vi "Setup4 Config.vi"(7 "Ring":u16(ring) items=["Read from ini files (to cluster Params)", "Write to ini file (from cluster Params)", "Copy ini file to new Path", "Create new lookup table by default value"], 8 "error in (no error)":errorcluster, 9 "Copy path":path, 10 "Config file to read/write":path, 11 "Params in":T2={"TaskIDs"={"DAQ tasks"={"Px taskID"=0, "Py taskID"=0, "Pz taskID"=0, "AOM taskID"=0, "Clock taskID"=0, "AI taskID"=0}, "DVEHandle"=refnum}, "Manual Control"={"Rotation Control"={"Phase"=0.0, "A amp (0-120)"=75.0, "B amp (0-120)"=53.3, "mean freq  [MHz]\ndefault 39.99"=40.0, "freq difference [Hz]"=2.0, "Enable A"=TRUE, "Enable B"=TRUE}, "X piezo\n [nm]"=0.0, "Y peizo\n [nm]"=0.0, "trap height\n [nm]"=5.012658227848101, "AOM0 \nPower"=0.2}, "Piezo Calibr"={"Px2Vx(AO)"=nan, "Py2Vy(AO)"=nan, "Pz2Vz(AO)"=nan, "Min Px"=nan, "Min Py"=nan, "Min Pz"=nan, "Max Px"=nan, "Max Py"=nan, "Max Pz"=nan, "Vx0 (V)"=nan, "Vy0 (V)"=nan, "Vz0 (V)"=nan}, "Instrument Calibr"={"Angular compensation coeffs"=[], "TetherCenter"={"TrapX_AO 0 [nm]"=nan, "TrapY_AO 0 [nm]"=nan, "TrapZ_AO 0 [nm]"=nan}, "XYZsignal baseline"={"Xsignal0"=nan, "Ysignal0"=nan, "Zsignal0"=nan, "Zsig slope"=nan, "Z bead0"=nan}, "S and P to Vs0"={"Vs0/P"=1.0, "Vs0/S"=1.0}, "Psi"=0.0, "ePS:eRL drift correlation"={"Interc P"=nan, "Slope P"=nan, "Interc S"=nan, "Slope S"=nan}, "Current piezo volt AO"={"Vpx_AO [V]"=nan, "Vpy_AO [V]"=nan, "Vpz_AO [V]"=nan}}, "Cylinder Calibr"={"ZStiff"=nan, "Zsens"=nan, "AngStiff"=nan, "XStiff"=nan, "Xsens"=nan, "MaxEllip"=nan, "YStiff"=nan, "Ysens"=nan, "FocalShift"=nan, "Sfz"=nan, "1/Sz"=nan, "Stau"=nan, "Sfx"=nan, "1/Sx"=nan, "1/Sang"=nan, "Sfy"=nan, "1/Sy"=nan, "1/focal"=nan, "ZsignalHeightDependence (1/nm)"=0.0}, "DAQParams"={"Buffer size"=nan, "Scanning rate"=nan, "Average"=nan, "Sampling rate"=nan, "set dt"=nan}, "DAQ channel offsets"={"A0 [V]"=0.0, "D0 [V]"=0.0, "P0  [V]"=0.0, "S0 [V]"=0.0, "L0 [V]"=0.0, "R0 [V]"=0.0, "Vpx0 [V]"=0.0, "Vpy0 [V]"=0.0, "Vpz0 [V]"=0.0, "Vsum0 [V]"=0.0, "Vpx_AO0 [V]"=0.0, "Vpy_AO0 [V]"=0.0, "Vpz_AO0 [V]"=0.0}, "Z bead polynomial coeffs"=[nan, nan, nan, nan], "Skip button ref"=refnum, "z bead lookup table"={"z signal"=[], "z bead"=[]}, "SP->power Matrix"=[], "Ms2p"=[], "Mp2s"=[], "Polynomial coeff V_px,y,z 2 position (nm)"=[]} {"Cylinder Calibr"."ZsignalHeightDependence (1/nm)" format="%.4e"; "Instrument Calibr"."Psi" format="%#_2f"; "Manual Control"."Y peizo\n [nm]" step=100.0 scale=0.0..30000.0; "Manual Control"."AOM0 \nPower" scale=0.0..1.0; "Manual Control"."X piezo\n [nm]" step=100.0 scale=0.0..30000.0; "Manual Control"."Rotation Control"."mean freq  [MHz]\ndefault 39.99" min=0.0 step=0.01; "Manual Control"."Rotation Control"."B amp (0-120)" min=0.0 max=120.0 step=0.1 format="%.1f"; "Manual Control"."Rotation Control"."A amp (0-120)" min=0.0 max=120.0 step=0.1 format="%.1f"; "Manual Control"."Rotation Control"."Phase" scale=0.0..360.0; "Manual Control"."trap height\n [nm]" scale=1000.0..7500.0; "TaskIDs"."DAQ tasks"."Px taskID" format="%x"; "TaskIDs"."DAQ tasks"."Py taskID" format="%x"; "TaskIDs"."DAQ tasks"."Pz taskID" format="%x"; "TaskIDs"."DAQ tasks"."AOM taskID" format="%x"; "TaskIDs"."DAQ tasks"."Clock taskID" format="%x"; "TaskIDs"."DAQ tasks"."AI taskID" format="%x"}) -> (0 "error out":errorcluster, 2 "file path out":path, 3 "Params out":T2={"TaskIDs"={"DAQ tasks"={"Px taskID"=0, "Py taskID"=0, "Pz taskID"=0, "AOM taskID"=0, "Clock taskID"=0, "AI taskID"=0}, "DVEHandle"=refnum}, "Manual Control"={"Rotation Control"={"Phase"=0.0, "A amp (0-120)"=75.0, "B amp (0-120)"=53.3, "mean freq  [MHz]\ndefault 39.99"=40.0, "freq difference [Hz]"=2.0, "Enable A"=TRUE, "Enable B"=TRUE}, "X piezo\n [nm]"=0.0, "Y peizo\n [nm]"=0.0, "trap height\n [nm]"=5.012658227848101, "AOM0 \nPower"=0.2}, "Piezo Calibr"={"Px2Vx(AO)"=nan, "Py2Vy(AO)"=nan, "Pz2Vz(AO)"=nan, "Min Px"=nan, "Min Py"=nan, "Min Pz"=nan, "Max Px"=nan, "Max Py"=nan, "Max Pz"=nan, "Vx0 (V)"=nan, "Vy0 (V)"=nan, "Vz0 (V)"=nan}, "Instrument Calibr"={"Angular compensation coeffs"=[], "TetherCenter"={"TrapX_AO 0 [nm]"=nan, "TrapY_AO 0 [nm]"=nan, "TrapZ_AO 0 [nm]"=nan}, "XYZsignal baseline"={"Xsignal0"=nan, "Ysignal0"=nan, "Zsignal0"=nan, "Zsig slope"=nan, "Z bead0"=nan}, "S and P to Vs0"={"Vs0/P"=1.0, "Vs0/S"=1.0}, "Psi"=0.0, "ePS:eRL drift correlation"={"Interc P"=nan, "Slope P"=nan, "Interc S"=nan, "Slope S"=nan}, "Current piezo volt AO"={"Vpx_AO [V]"=nan, "Vpy_AO [V]"=nan, "Vpz_AO [V]"=nan}}, "Cylinder Calibr"={"ZStiff"=nan, "Zsens"=nan, "AngStiff"=nan, "XStiff"=nan, "Xsens"=nan, "MaxEllip"=nan, "YStiff"=nan, "Ysens"=nan, "FocalShift"=nan, "Sfz"=nan, "1/Sz"=nan, "Stau"=nan, "Sfx"=nan, "1/Sx"=nan, "1/Sang"=nan, "Sfy"=nan, "1/Sy"=nan, "1/focal"=nan, "ZsignalHeightDependence (1/nm)"=0.0}, "DAQParams"={"Buffer size"=nan, "Scanning rate"=nan, "Average"=nan, "Sampling rate"=nan, "set dt"=nan}, "DAQ channel offsets"={"A0 [V]"=0.0, "D0 [V]"=0.0, "P0  [V]"=0.0, "S0 [V]"=0.0, "L0 [V]"=0.0, "R0 [V]"=0.0, "Vpx0 [V]"=0.0, "Vpy0 [V]"=0.0, "Vpz0 [V]"=0.0, "Vsum0 [V]"=0.0, "Vpx_AO0 [V]"=0.0, "Vpy_AO0 [V]"=0.0, "Vpz_AO0 [V]"=0.0}, "Z bead polynomial coeffs"=[nan, nan, nan, nan], "Skip button ref"=refnum, "z bead lookup table"={"z signal"=[], "z bead"=[]}, "SP->power Matrix"=[], "Ms2p"=[], "Mp2s"=[], "Polynomial coeff V_px,y,z 2 position (nm)"=[]} {"Cylinder Calibr"."ZsignalHeightDependence (1/nm)" format="%.4e"; "Instrument Calibr"."Psi" format="%#_2f"; "Manual Control"."Y peizo\n [nm]" step=100.0 scale=0.0..30000.0; "Manual Control"."AOM0 \nPower" scale=0.0..1.0; "Manual Control"."X piezo\n [nm]" step=100.0 scale=0.0..30000.0; "Manual Control"."Rotation Control"."mean freq  [MHz]\ndefault 39.99" min=0.0 step=0.01; "Manual Control"."Rotation Control"."B amp (0-120)" min=0.0 max=120.0 step=0.1 format="%.1f"; "Manual Control"."Rotation Control"."A amp (0-120)" min=0.0 max=120.0 step=0.1 format="%.1f"; "Manual Control"."Rotation Control"."Phase" scale=0.0..360.0; "Manual Control"."trap height\n [nm]" scale=1000.0..7500.0; "TaskIDs"."DAQ tasks"."Px taskID" format="%x"; "TaskIDs"."DAQ tasks"."Py taskID" format="%x"; "TaskIDs"."DAQ tasks"."Pz taskID" format="%x"; "TaskIDs"."DAQ tasks"."AOM taskID" format="%x"; "TaskIDs"."DAQ tasks"."Clock taskID" format="%x"; "TaskIDs"."DAQ tasks"."AI taskID" format="%x"})   [LabVIEW 2020, in "Initialization.lvlib" / "FileManagement.lvlib"]
uses:
  FileManagement.lvlib
  Param.ctl
  ManualCtrl.ctl
  DVESetting.ctl
  CylinderCalibrNew.ctl
  SignalConversion/DAQChannelOffsets.ctl
  <vilib>/Analysis/Matrix/Datatypes/RealMatrix.ctl
  configuration file sections, keys and values.ctl
  <vilib>/Utility/config.llb/Read Key (Double).vi
  <vilib>/Utility/config.llb/Read Key (String).vi
  <vilib>/Utility/config.llb/Read Key (I32).vi
  <vilib>/Analysis/baseanly.llb/Real Inverse Matrix.vi
  <vilib>/Utility/config.llb/Write Key (Double).vi
  <vilib>/Utility/config.llb/Write Key (String).vi
  <vilib>/Utility/config.llb/NI_LVConfig.lvlib
  <vilib>/Analysis/NI_AALBase.lvlib
  Initialization.lvlib
  <vilib>/Analysis/Matrix/NI_Matrix.lvlib
  SignalConversion/SignalConverson.lvlib
panel:
  in  "Piezo sensor conversion coeffs key":string="AI2p"
  out "transposed array":dbl[][](array[numeric])
  out "look up table check":string
  in  "configuration file sections, keys and values":T1={"Section 1"="Trap and cylinder calibration", "Keys of Section 1"=["Kz, pN/nm/W", "Kx, pN/nm/W", "Ky, pN/nm/W", "Sz, 1/nm", "Sx, 1/nm", "Sy, 1/nm", "Kang, pNnm/rad/W", "Max ellipticity, 1", "Focal shift", "ZsignalHeightDependence, 1/nm"], "Values (read) of Section 1"=[0.468, 4.584, 4.884, 0.000564, 0.001578, 0.00166, 30700.0, 0.0204, 0.75, 6.2e-07], "Section 2"="Piezo AO calibration and settings", "Keys of Section 2"=["Vx/Px(V/nm)", "Vy/Py(V/nm)", "Vz/Pz(V/nm)", "Max Px (nm)", "Max Py (nm)", "Max Pz (nm)", "Min Px (nm)", "Min Py (nm)", "Min Pz (nm)", "Vx0 (V)", "Vy0 (V)", "Vz0 (V)"], "Values (read) of Section 2"=[0.000665, 0.000665, 0.002, 10000.0, 10000.0, 10000.0, 0.0, 0.0, 0.0, -10.0, -10.0, -10.0], "Section 3"="matrix Mp2s (3X3)", "Keys of Section 3"=["a11", "a12", "a13", "a21", "a22", "a23", "a31", "a32", "a33"], "Values (read) of Section 3"=[1.0, 0.0, 0.0, 0.0, 1.0, 0.0, 0.0, 0.198, 1.0], "Section 4"="DAQ settings", "Keys of Section 4"=["AIBufferSize", "DAQ ScanRate", "Points to average", "Samping rate"], "Values (read) of Section 4"=[100000, 10000, 20, 500], "Section 5"="PS detector signal to laser power (W) conversion matrix (2X2)", "Keys of Section 5"=["a11", "a12", "a21", "a22"], "Values (read) of Section 5"=[-0.018123, 0.000111, 4.2e-05, -0.018644], "Section 6"="Z bead vs Z signal polynomial coefficients (nm)", "Keys of Section 6"=["a0", "a1", "a2", "a3", "a4", "a5"], "Values (read) of Section 6"=[0.0, 1064.07, 1642.745, 6870.906, -346812.49, 1661133.202], "Section 7"="Z bead look up table", "Keys of Section 7"=["(Z signal, Z bead)"], "Values (read) of Section 7"=[]}
  out "succeeded in writing to ini file ?":bool
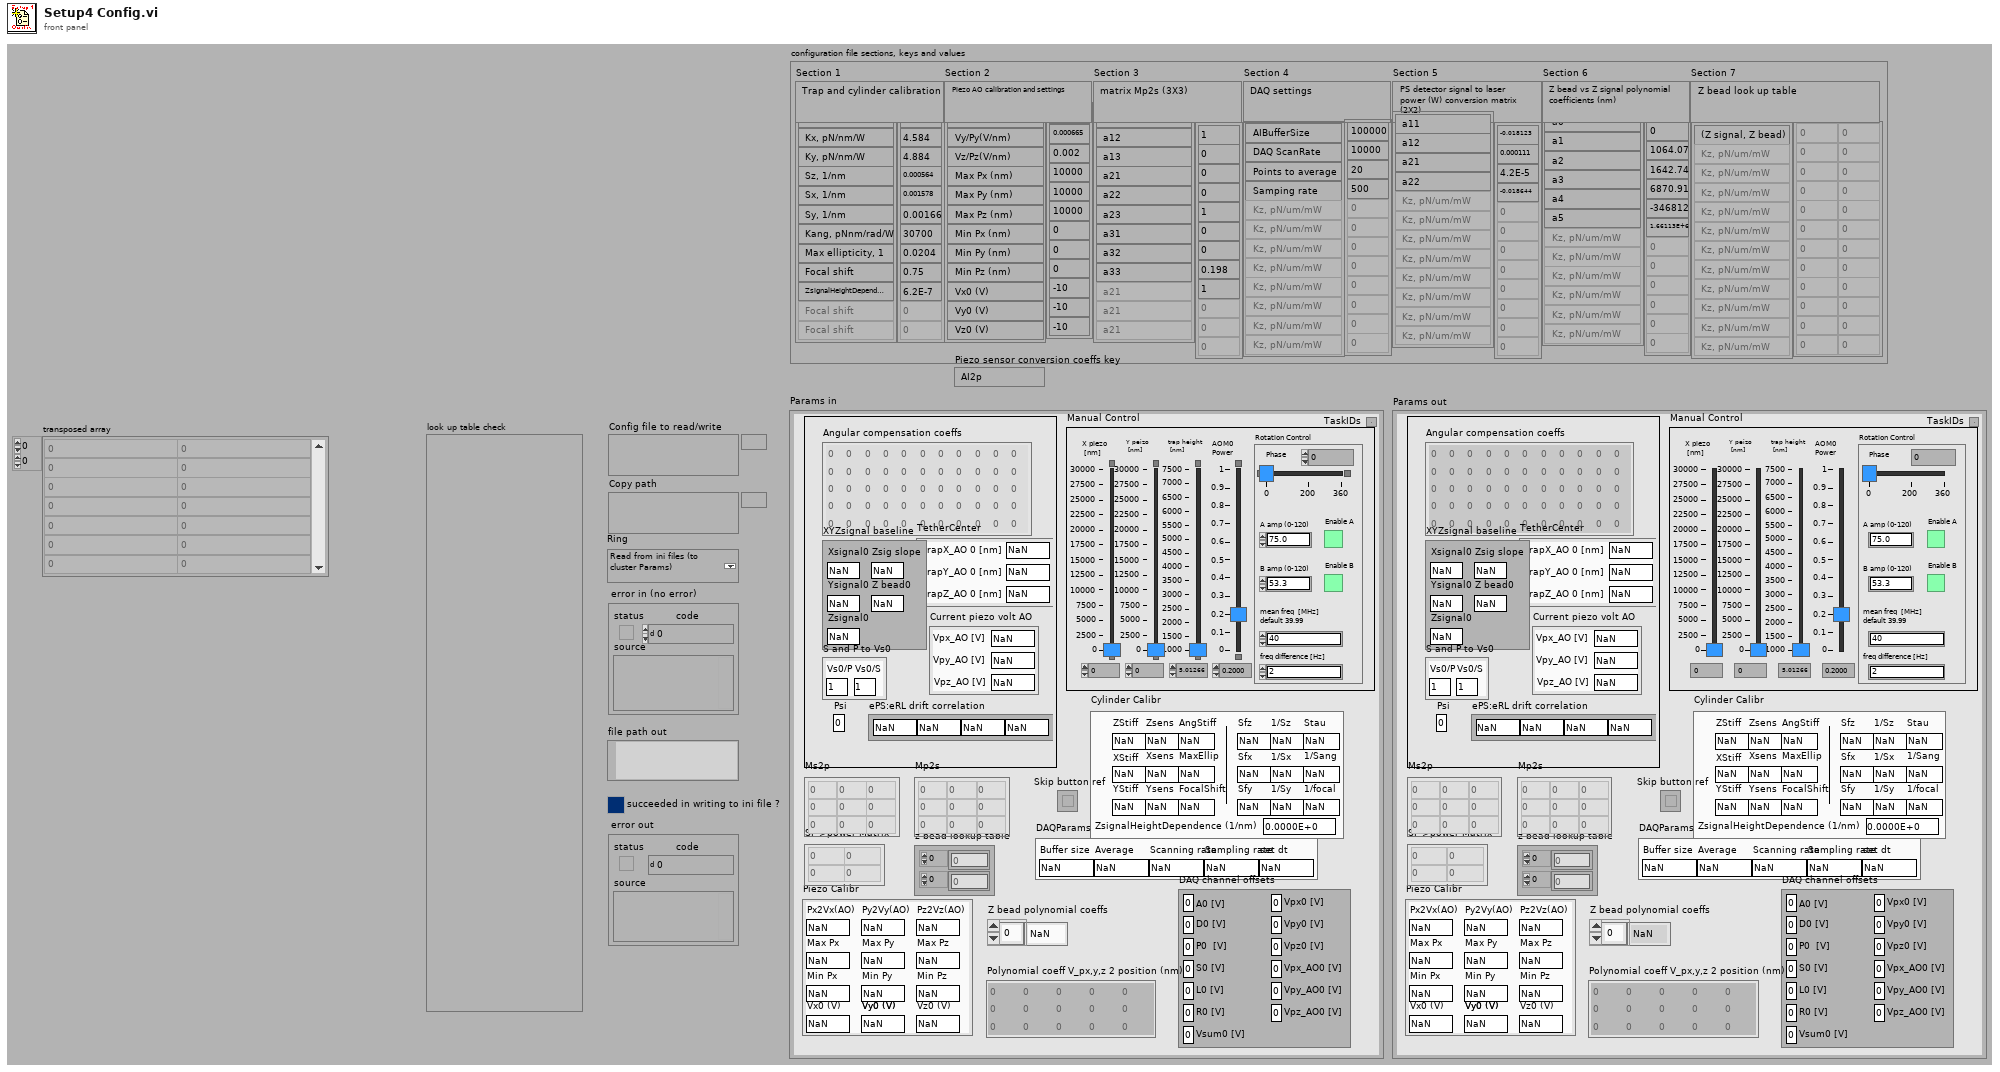
[diagram p1: front panel]
types:
  T1 = typedef "Initialization.lvlib/FileManagement.lvlib/configuration file sections, keys and values.ctl" = cluster{"Section 1":string, "Keys of Section 1":string[], "Values (read) of Section 1":dbl[], "Section 2":string, "Keys of Section 2":string[], "Values (read) of Section 2":dbl[], "Section 3":string, "Keys of Section 3":string[], "Values (read) of Section 3":dbl[], "Section 4":string, "Keys of Section 4":string[], "Values (read) of Section 4":i32[], "Section 5":string, "Keys of Section 5":string[], "Values (read) of Section 5":dbl[], "Section 6":string, "Keys of Section 6":string[], "Values (read) of Section 6":dbl[], "Section 7":string, "Keys of Section 7":string[], "Values (read) of Section 7":dbl[][]}
  T2 = typedef "Initialization.lvlib/Param.ctl" = cluster{"TaskIDs":cluster{"DAQ tasks":cluster{"Px taskID":u32, "Py taskID":u32, "Pz taskID":u32, "AOM taskID":u32, "Clock taskID":u32, "AI taskID":u32}, "DVEHandle":refnum<file>}, "Manual Control":T3, "Piezo Calibr":cluster{"Px2Vx(AO)":dbl, "Py2Vy(AO)":dbl, "Pz2Vz(AO)":dbl, "Min Px":dbl, "Min Py":dbl, "Min Pz":dbl, "Max Px":dbl, "Max Py":dbl, "Max Pz":dbl, "Vx0 (V)":dbl, "Vy0 (V)":dbl, "Vz0 (V)":dbl}, "Instrument Calibr":cluster{"Angular compensation coeffs":dbl[][], "TetherCenter":cluster{"TrapX_AO 0 [nm]":dbl, "TrapY_AO 0 [nm]":dbl, "TrapZ_AO 0 [nm]":dbl}, "XYZsignal baseline":cluster{"Xsignal0":dbl, "Ysignal0":dbl, "Zsignal0":dbl, "Zsig slope":dbl, "Z bead0":dbl}, "S and P to Vs0":cluster{"Vs0/P":dbl, "Vs0/S":dbl}, "Psi":dbl, "ePS:eRL drift correlation":cluster{"Interc P":dbl, "Slope P":dbl, "Interc S":dbl, "Slope S":dbl}, "Current piezo volt AO":cluster{"Vpx_AO [V]":dbl, "Vpy_AO [V]":dbl, "Vpz_AO [V]":dbl}}, "Cylinder Calibr":T5, "DAQParams":cluster{"Buffer size":dbl, "Scanning rate":dbl, "Average":dbl, "Sampling rate":dbl, "set dt":dbl}, "DAQ channel offsets":T6, "Z bead polynomial coeffs":dbl[], "Skip button ref":refnum<vi>, "z bead lookup table":cluster{"z signal":dbl[], "z bead":dbl[]}, "SP->power Matrix":T7, "Ms2p":T7, "Mp2s":T7, "Polynomial coeff V_px,y,z 2 position (nm)":dbl[][]}
  T3 = typedef "Initialization.lvlib/ManualCtrl.ctl" = cluster{"Rotation Control":T4, "X piezo\n [nm]":dbl, "Y peizo\n [nm]":dbl, "trap height\n [nm]":dbl, "AOM0 \nPower":dbl}
  T4 = typedef "Initialization.lvlib/DVESetting.ctl" = cluster{"Phase":dbl, "A amp (0-120)":dbl, "B amp (0-120)":dbl, "mean freq  [MHz]\ndefault 39.99":dbl, "freq difference [Hz]":dbl, "Enable A":bool, "Enable B":bool}
  T5 = typedef "Initialization.lvlib/CylinderCalibrNew.ctl" = cluster{"ZStiff":dbl, "Zsens":dbl, "AngStiff":dbl, "XStiff":dbl, "Xsens":dbl, "MaxEllip":dbl, "YStiff":dbl, "Ysens":dbl, "FocalShift":dbl, "Sfz":dbl, "1/Sz":dbl, "Stau":dbl, "Sfx":dbl, "1/Sx":dbl, "1/Sang":dbl, "Sfy":dbl, "1/Sy":dbl, "1/focal":dbl, "ZsignalHeightDependence (1/nm)":dbl}
  T6 = typedef "SignalConverson.lvlib/DAQChannelOffsets.ctl" = cluster{"A0 [V]":dbl, "D0 [V]":dbl, "P0  [V]":dbl, "S0 [V]":dbl, "L0 [V]":dbl, "R0 [V]":dbl, "Vpx0 [V]":dbl, "Vpy0 [V]":dbl, "Vpz0 [V]":dbl, "Vsum0 [V]":dbl, "Vpx_AO0 [V]":dbl, "Vpy_AO0 [V]":dbl, "Vpz_AO0 [V]":dbl}
  T7 = typedef "NI_Matrix.lvlib/RealMatrix.ctl" = dbl[][]
  T8 = typedef "NI_LVConfig.lvlib/Config Data RefNum.ctl" = refnum<k1>
  T9 = cluster{"Px2Vx(AO)":dbl, "Py2Vy(AO)":dbl, "Pz2Vz(AO)":dbl, "Min Px":dbl, "Min Py":dbl, "Min Pz":dbl, "Max Px":dbl, "Max Py":dbl, "Max Pz":dbl, "Vx0 (V)":dbl, "Vy0 (V)":dbl, "Vz0 (V)":dbl}
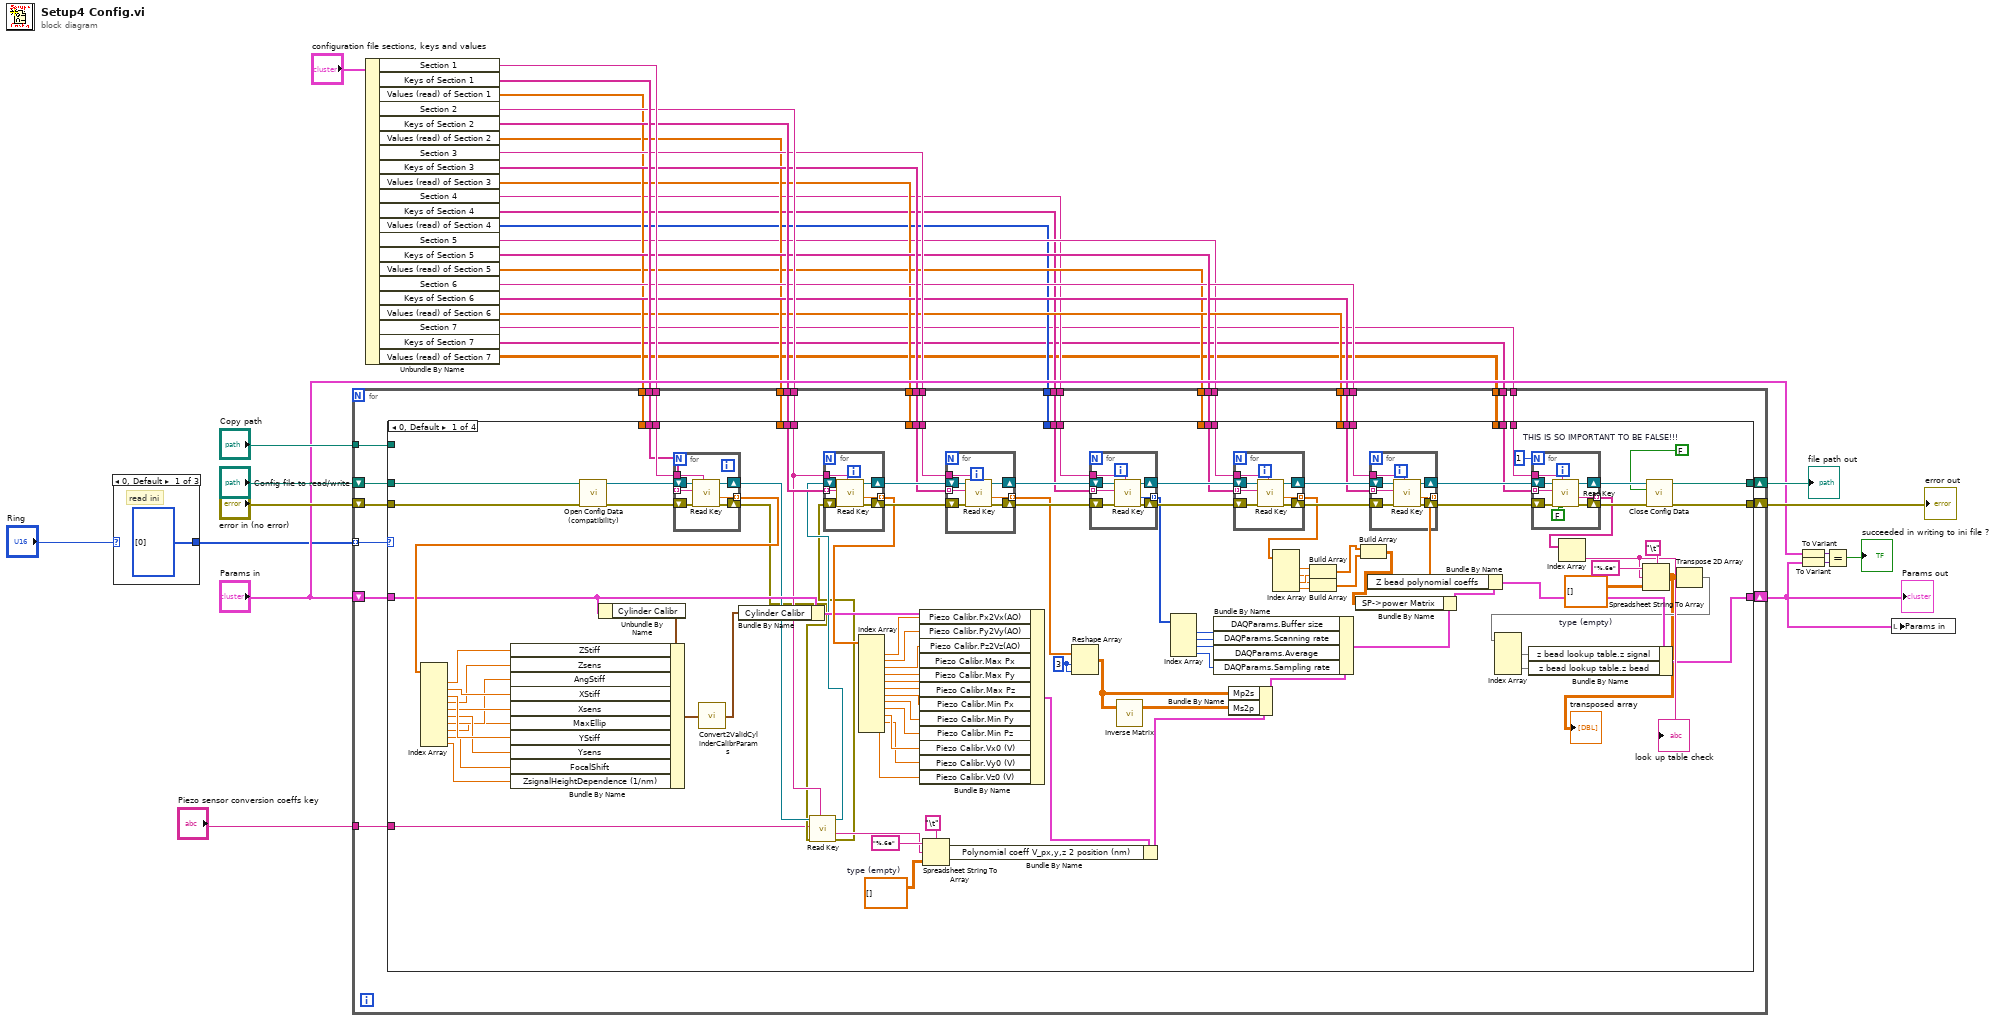
[diagram p0: block diagram]
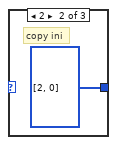
[diagram p2: hidden frame]
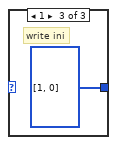
[diagram p3: hidden frame]
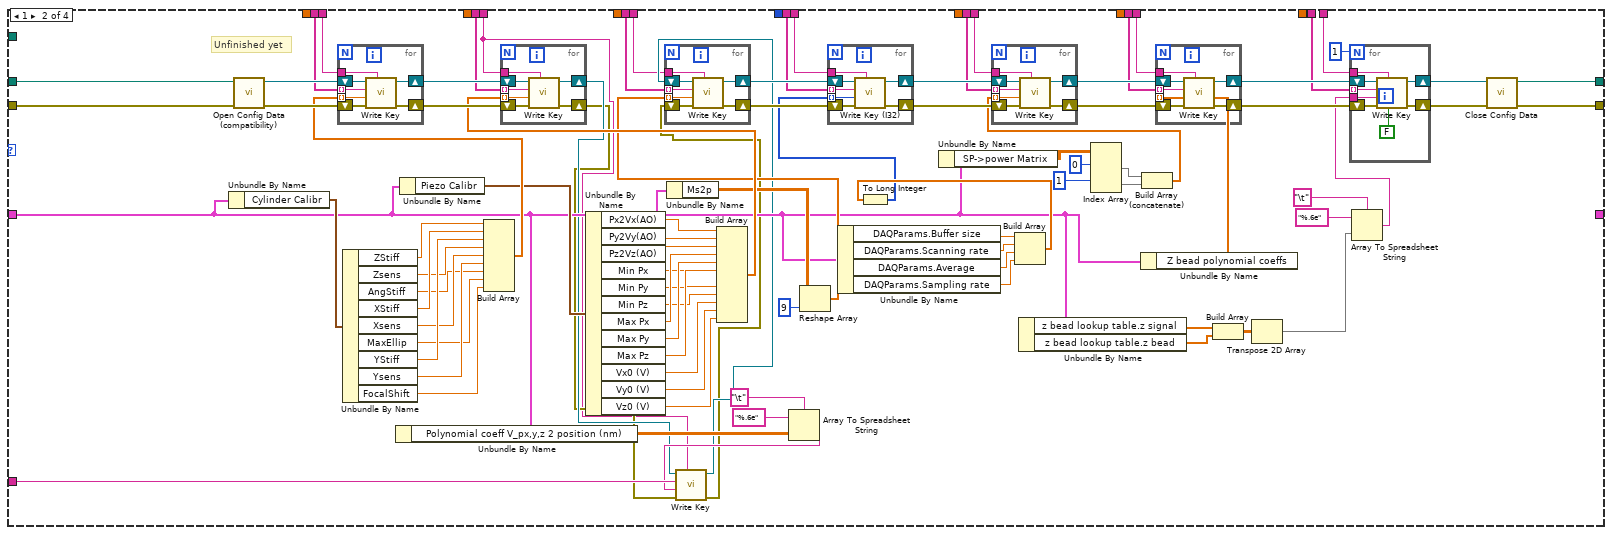
[diagram p4: hidden frame]
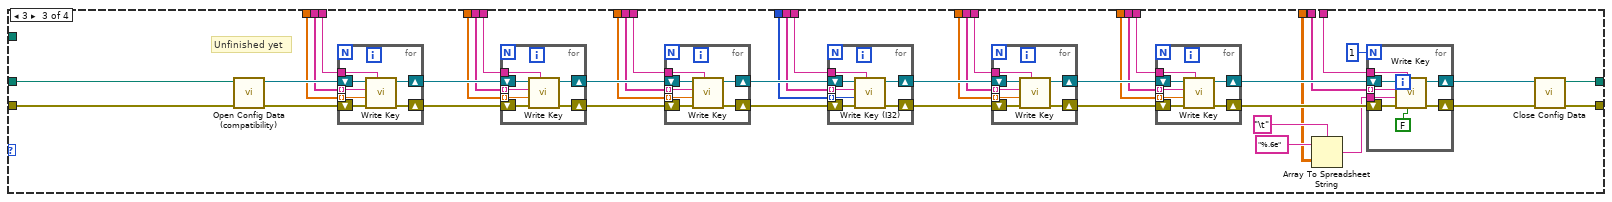
[diagram p5: hidden frame]
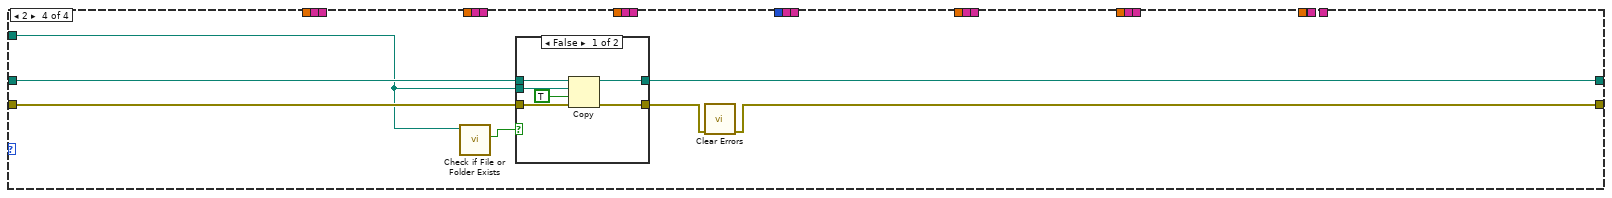
[diagram p6: hidden frame]
diagram:
  n1 = case shown="0, Default" "Ring" {
    tunnel: [i32[] [0] i32[] [2, 0] i32[] [1, 0]] -> w25
    frame 0, Default {
      # "read ini"
    }
    frame 2 {
      # "copy ini"
    }
    frame 1 {
      # "write ini"
    }
  }
  n2 = Unbundle By Name("configuration file sections, keys and values") -> ("Section 1"=w23:string, "Keys of Section 1"=w22:string[], "Values (read) of Section 1"=w14:dbl[], "Section 2"=w21:string, "Keys of Section 2"=w20:string[], "Values (read) of Section 2"=w13:dbl[], "Section 3"=w19:string, "Keys of Section 3"=w18:string[], "Values (read) of Section 3"=w12:dbl[], "Section 4"=w6:string, "Keys of Section 4"=w7:string[], "Values (read) of Section 4"=w8:i32[], "Section 5"=w9:string, "Keys of Section 5"=w17:string[], "Values (read) of Section 5"=w10:dbl[], "Section 6"=w16:string, "Keys of Section 6"=w15:string[], "Values (read) of Section 6"=w11:dbl[], "Section 7"=w5:string, "Keys of Section 7"=w4:string[], "Values (read) of Section 7"=w3:dbl[][])
  n3 = for {
    tunnel: w25 -> [w66] mode=indexing
    tunnel: w23 -> [w64]
    tunnel: w22 -> [w63]
    tunnel: w20 -> [w62]
    tunnel: w21 -> [w61]
    tunnel: w18 -> [w60]
    tunnel: w19 -> [w59]
    tunnel: w6 -> [w58]
    tunnel: w7 -> [w57]
    tunnel: w17 -> [w56]
    tunnel: w9 -> [w55]
    tunnel: w16 -> [w54]
    tunnel: w15 -> [w53]
    tunnel: "Copy path" -> [w51]
    shift-right: [w52] -> w32
    shift-left: "Config file to read/write" -> [w68]
    shift-right: [w65] -> w33
    shift-left: "error in (no error)" -> [w67]
    shift-right: [w49] -> w1
    shift-left: "Params in" -> [w50]
    tunnel: w14 -> [w48]
    tunnel: w13 -> [w47]
    tunnel: w12 -> [w46]
    tunnel: w8 -> [w45]
    tunnel: w10 -> [w44]
    tunnel: w11 -> [w43]
    tunnel: w5 -> [w42]
    tunnel: w4 -> [w41]
    tunnel: w3 -> [w40]
    tunnel: "Piezo sensor conversion coeffs key" -> [w39]
    n4 = case shown="0, Default" w66 {
      tunnel: w68 -> [w175 w316 w411 w468]
      tunnel: w67 -> [w174 w315 w410 w466]
      tunnel: [w87 w312 w407 w464] -> w65
      tunnel: w64 -> [w171 w311 w406 _]
      tunnel: w63 -> [w170 w310 w405 _]
      tunnel: w62 -> [w169 w307 w402 _]
      tunnel: w61 -> [w85 w226 w401 _]
      tunnel: w60 -> [w166 w306 w398 _]
      tunnel: w59 -> [w165 w227 w397 _]
      tunnel: w58 -> [w162 w303 w394 _]
      tunnel: w57 -> [w161 w302 w393 _]
      tunnel: w56 -> [w158 w299 w390 _]
      tunnel: w55 -> [w157 w298 w389 _]
      tunnel: w54 -> [w154 w295 w386 _]
      tunnel: w53 -> [w153 w294 w385 _]
      tunnel: [w152 w293 w384 w467] -> w52
      tunnel: w51 -> [_ _ _ w463]
      tunnel: w50 -> [w115 w235 _ _]
      tunnel: [w100 _ _ _] -> w49
      tunnel: w48 -> [_ _ w383 _]
      tunnel: w47 -> [_ _ w382 _]
      tunnel: w46 -> [_ _ w381 _]
      tunnel: w45 -> [_ _ w380 _]
      tunnel: w44 -> [_ _ w379 _]
      tunnel: w43 -> [_ _ w378 _]
      tunnel: w42 -> [w109 w256 w373 _]
      tunnel: w41 -> [w108 w255 w372 _]
      tunnel: w40 -> [_ _ w369 _]
      tunnel: w39 -> [w70 w233 _ _]
      frame 0, Default {
        w79 = dbl[][] []  # type (empty)
        w104 = dbl[][] []  # type (empty)
        w86 = FALSE  # THIS IS SO IMPORTANT TO BE FALSE!!!
        w127 = 3 ("dimension size")
        n5 = call <vilib>:"Open Config Data (compatibility).vi"("error in (no error)"=w174, "configuration file path"=w175) -> ("error out"=w173:errorcluster, "refnum"=w172:T8)  [unwired: 7 in, 1 out]
        n6 = Unbundle By Name(w115) -> ("Cylinder Calibr"=w141:T5)
        n7 = for {
          tunnel: w171 -> [w221]
          tunnel: w170 -> [w220] mode=indexing
          shift-right: [w222] -> w74
          shift-left: w172 -> [w224]
          shift-right: [w223] -> w72
          shift-left: w173 -> [w225]
          tunnel: [w219] -> w150 mode=indexing
          n8 = call-poly <vilib>:"Read Key.vi"("section"=w221, "error in (no error)"=w225, "key"=w220, "refnum"=w224) -> ("error out"=w223:errorcluster, "value"=w219:dbl, "refnum out"=w222:T8)  [unwired: 4 in, 1 out]
        }
        n9 = Index Array(array=w150) -> (element #1=w140:dbl, element #2=w149:dbl, element #3=w148:dbl, element #4=w147:dbl, element #5=w146:dbl, element #6=w145:dbl, element #7=w144:dbl, element #8=w143:dbl, element #9=w142:dbl, element #10=w69:dbl)  [unwired: 10 in]
        n10 = Bundle By Name(cluster=w141, "ZStiff"=w140, "Zsens"=w147, "AngStiff"=w144, "XStiff"=w149, "Xsens"=w146, "MaxEllip"=w143, "YStiff"=w148, "Ysens"=w145, "FocalShift"=w142, "ZsignalHeightDependence (1/nm)"=w69) -> (w139:T5)
        n11 = call "Convert2ValidCylinderCalibrParams.vi"("CylinderCalibrNew in"=w139) -> ("CylinderCalibrNew out"=w151:T5)
        n12 = Bundle By Name(cluster=w115, "Cylinder Calibr"=w151) -> (w114:T2)
        n13 = call-poly <vilib>:"Read Key.vi"("section"=w85, "error in (no error)"=w72, "key"=w70, "refnum"=w74) -> ("error out"=w71:errorcluster, "value"=w78:string, "refnum out"=w73:T8)  [unwired: 4 in, 1 out]
        n14 = for {
          tunnel: w85 -> [w214]
          tunnel: w169 -> [w213] mode=indexing
          shift-right: [w215] -> w167
          shift-left: w73 -> [w217]
          shift-right: [w216] -> w168
          shift-left: w71 -> [w218]
          tunnel: [w212] -> w138 mode=indexing
          n15 = call-poly <vilib>:"Read Key.vi"("section"=w214, "error in (no error)"=w218, "key"=w213, "refnum"=w217) -> ("error out"=w216:errorcluster, "value"=w212:dbl, "refnum out"=w215:T8)  [unwired: 4 in, 1 out]
        }
        n16 = Index Array(array=w138) -> (element #1=w137:dbl, element #2=w136:dbl, element #3=w135:dbl, element #4=w134:dbl, element #5=w133:dbl, element #6=w132:dbl, element #7=w131:dbl, element #8=w130:dbl, element #9=w129:dbl, element #10=w84:dbl, element #11=w83:dbl, element #12=w82:dbl)  [unwired: 12 in]
        n17 = Bundle By Name(cluster=w114, "Piezo Calibr.Px2Vx(AO)"=w137, "Piezo Calibr.Py2Vy(AO)"=w136, "Piezo Calibr.Pz2Vz(AO)"=w135, "Piezo Calibr.Max Px"=w134, "Piezo Calibr.Max Py"=w133, "Piezo Calibr.Max Pz"=w132, "Piezo Calibr.Min Px"=w131, "Piezo Calibr.Min Py"=w130, "Piezo Calibr.Min Pz"=w129, "Piezo Calibr.Vx0 (V)"=w84, "Piezo Calibr.Vy0 (V)"=w83, "Piezo Calibr.Vz0 (V)"=w82) -> (w76:T2)
        n18 = Spreadsheet String To Array(delimiter (Tab)="\t" ("delimiter (\\t)"), format string="%.6e" ("format (%.6e)"), spreadsheet string=w78, array type (2D Dbl)=w79) -> (array=w77:dbl[][])
        n19 = for {
          tunnel: w165 -> [w207]
          tunnel: w166 -> [w206] mode=indexing
          shift-right: [w208] -> w163
          shift-left: w167 -> [w210]
          shift-right: [w209] -> w164
          shift-left: w168 -> [w211]
          tunnel: [w205] -> w126 mode=indexing
          n20 = call-poly <vilib>:"Read Key.vi"("section"=w207, "error in (no error)"=w211, "key"=w206, "refnum"=w210) -> ("error out"=w209:errorcluster, "value"=w205:dbl, "refnum out"=w208:T8)  [unwired: 4 in, 1 out]
        }
        n21 = Bundle By Name(cluster=w76, "Polynomial coeff V_px,y,z 2 position (nm)"=w77) -> (w75:T2)
        n22 = Reshape Array(w126, w127, w127) -> (w125:dbl[][])
        n23 = for {
          tunnel: w162 -> [w200]
          tunnel: w161 -> [w199] mode=indexing
          shift-right: [w201] -> w160
          shift-left: w163 -> [w203]
          shift-right: [w202] -> w159
          shift-left: w164 -> [w204]
          tunnel: [w198] -> w123 mode=indexing
          n24 = call-poly <vilib>:"Read Key.vi"("section"=w200, "error in (no error)"=w204, "key"=w199, "refnum"=w203) -> ("error out"=w202:errorcluster, "value"=w198:i32, "refnum out"=w201:T8)  [unwired: 4 in, 1 out]
        }
        n25 = call-poly <vilib>:"Inverse Matrix.vi"("Input Matrix"=w125) -> ("Inverse Matrix"=w128:T7)  [unwired: 1 in, 1 out]
        n26 = Index Array(array=w123) -> (element #1=w122:i32, element #2=w121:i32, element #3=w120:i32, element #4=w119:i32)  [unwired: 4 in]
        n27 = Bundle By Name(cluster=w75, "Mp2s"=w125, "Ms2p"=w128) -> (w124:T2)
        n28 = Bundle By Name(cluster=w124, "DAQParams.Buffer size"=w122, "DAQParams.Scanning rate"=w121, "DAQParams.Average"=w120, "DAQParams.Sampling rate"=w119) -> (w118:T2)
        n29 = for {
          tunnel: w157 -> [w193]
          tunnel: w158 -> [w192] mode=indexing
          shift-right: [w194] -> w156
          shift-left: w160 -> [w196]
          shift-right: [w195] -> w155
          shift-left: w159 -> [w197]
          tunnel: [w191] -> w95 mode=indexing
          n30 = call-poly <vilib>:"Read Key.vi"("section"=w193, "error in (no error)"=w197, "key"=w192, "refnum"=w196) -> ("error out"=w195:errorcluster, "value"=w191:dbl, "refnum out"=w194:T8)  [unwired: 4 in, 1 out]
        }
        n31 = Index Array(array=w95) -> (element #1=w94:dbl, element #2=w92:dbl, element #3=w93:dbl, element #4=w91:dbl)  [unwired: 4 in]
        n32 = Build Array(w94, w93) -> (w90:dbl[])
        n33 = Build Array(w92, w91) -> (w89:dbl[])
        n34 = Build Array(w90, w89) -> (w88:dbl[][])
        n35 = Bundle By Name(cluster=w118, "SP->power Matrix"=w88) -> (w117:T2)
        n36 = for {
          tunnel: w154 -> [w186]
          tunnel: w153 -> [w185] mode=indexing
          shift-right: [w187] -> w113
          shift-left: w156 -> [w189]
          shift-right: [w188] -> w112
          shift-left: w155 -> [w190]
          tunnel: [w184] -> w116 mode=indexing
          n37 = call-poly <vilib>:"Read Key.vi"("section"=w186, "error in (no error)"=w190, "key"=w185, "refnum"=w189) -> ("error out"=w188:errorcluster, "value"=w184:dbl, "refnum out"=w187:T8)  [unwired: 4 in, 1 out]
        }
        n38 = Bundle By Name(cluster=w117, "Z bead polynomial coeffs"=w116) -> (w101:T2)
        n39 = for {
          N: 1 -> [_]
          tunnel: w109 -> [w179]
          tunnel: w108 -> [w178] mode=indexing
          shift-right: [w180] -> w111
          shift-left: w113 -> [w182]
          shift-right: [w181] -> w110
          shift-left: w112 -> [w183]
          tunnel: [w177] -> w103 mode=indexing
          n40 = call-poly <vilib>:"Read Key.vi"("read raw string? (F)"=FALSE, "section"=w179, "error in (no error)"=w183, "key"=w178, "refnum"=w182) -> ("error out"=w181:errorcluster, "value"=w177:string, "refnum out"=w180:T8)  [unwired: 3 in, 1 out]
        }
        n41 = Index Array(array=w103) -> (element=w102:string)  [unwired: 1 in]
        "look up table check" <- w102
        n42 = Spreadsheet String To Array(delimiter (Tab)="\t" ("delimiter (\\t)"), format string="%.6e" ("format (%.6e)"), spreadsheet string=w102, array type (2D Dbl)=w104) -> (array=w96:dbl[][])
        "transposed array" <- w96
        n43 = call <vilib>:"Close Config Data.vi"("error in (no error)"=w110, "write file if changed (T)"=w86, "refnum"=w111) -> ("error out"=w87:errorcluster, "file path"=w152:path)  [unwired: 7 in]
        n44 = Transpose 2D Array(2D array=w96) -> (transposed array=w99:dbl[][])
        n45 = Index Array(array=w99) -> (element #1=w98:dbl[], element #2=w97:dbl[])  [unwired: 4 in]
        n46 = Bundle By Name(cluster=w101, "z bead lookup table.z signal"=w98, "z bead lookup table.z bead"=w97) -> (w100:T2)
      }
      frame 1 {
        # "Unfinished yet"
        n47 = Unbundle By Name(w235) -> ("Cylinder Calibr"=w292:T5)
        n48 = call <vilib>:"Open Config Data (compatibility).vi"("error in (no error)"=w315, "configuration file path"=w316) -> ("error out"=w314:errorcluster, "refnum"=w313:T8)  [unwired: 7 in, 1 out]
        n49 = Unbundle By Name(w292) -> ("ZStiff"=w291:dbl, "Zsens"=w288:dbl, "AngStiff"=w285:dbl, "XStiff"=w290:dbl, "Xsens"=w287:dbl, "MaxEllip"=w284:dbl, "YStiff"=w289:dbl, "Ysens"=w286:dbl, "FocalShift"=w283:dbl)
        n50 = Unbundle By Name(w235) -> ("Polynomial coeff V_px,y,z 2 position (nm)"=w234:dbl[][])
        n51 = Unbundle By Name(w235) -> ("Piezo Calibr"=w281:T9)
        n52 = Build Array(w291, w290, w289, w288, w287, w286, w285, w284, w283) -> (w282:dbl[])
        n53 = for {
          tunnel: w282 -> [w366] mode=indexing
          tunnel: w311 -> [w361]
          tunnel: w310 -> [w360] mode=indexing
          shift-right: [w362] -> w309
          shift-left: w313 -> [w364]
          shift-right: [w363] -> w308
          shift-left: w314 -> [w365]
          n54 = call-poly <vilib>:"Write Key.vi"("section"=w361, "error in (no error)"=w365, "value"=w366, "key"=w360, "refnum"=w364) -> ("error out"=w363:errorcluster, "refnum out"=w362:T8)  [unwired: 4 in, 1 out]
        }
        n55 = Unbundle By Name(w281) -> ("Px2Vx(AO)"=w280:dbl, "Py2Vy(AO)"=w279:dbl, "Pz2Vz(AO)"=w278:dbl, "Min Px"=w274:dbl, "Min Py"=w273:dbl, "Min Pz"=w272:dbl, "Max Px"=w277:dbl, "Max Py"=w276:dbl, "Max Pz"=w275:dbl, "Vx0 (V)"=w239:dbl, "Vy0 (V)"=w238:dbl, "Vz0 (V)"=w237:dbl)
        n56 = Unbundle By Name(w235) -> ("Ms2p"=w270:T7)
        n57 = Build Array(w280, w279, w278, w277, w276, w275, w274, w273, w272, w239, w238, w237) -> (w271:dbl[])
        n58 = for {
          tunnel: w271 -> [w359] mode=indexing
          tunnel: w226 -> [w354]
          tunnel: w307 -> [w353] mode=indexing
          shift-right: [w355] -> w231
          shift-left: w309 -> [w357]
          shift-right: [w356] -> w229
          shift-left: w308 -> [w358]
          n59 = call-poly <vilib>:"Write Key.vi"("section"=w354, "error in (no error)"=w358, "value"=w359, "key"=w353, "refnum"=w357) -> ("error out"=w356:errorcluster, "refnum out"=w355:T8)  [unwired: 4 in, 1 out]
        }
        n60 = Array To Spreadsheet String(delimiter (Tab)="\t" ("delimiter (\\t)"), array=w234, 3:"%.6e" ("format (%.3f)")) -> (spreadsheet string=w232:string)
        n61 = call-poly <vilib>:"Write Key.vi"("section"=w226, "error in (no error)"=w229, "value"=w232, "key"=w233, "refnum"=w231) -> ("error out"=w228:errorcluster, "refnum out"=w230:T8)  [unwired: 4 in, 1 out]
        n62 = Reshape Array(w270, 9 ("dimension size")) -> (w268:dbl[])
        n63 = for {
          tunnel: w268 -> [w352] mode=indexing
          tunnel: w227 -> [w347]
          tunnel: w306 -> [w346] mode=indexing
          shift-right: [w348] -> w304
          shift-left: w230 -> [w350]
          shift-right: [w349] -> w305
          shift-left: w228 -> [w351]
          n64 = call-poly <vilib>:"Write Key.vi"("section"=w347, "error in (no error)"=w351, "value"=w352, "key"=w346, "refnum"=w350) -> ("error out"=w349:errorcluster, "refnum out"=w348:T8)  [unwired: 4 in, 1 out]
        }
        n65 = Unbundle By Name(w235) -> ("DAQParams.Buffer size"=w267:dbl, "DAQParams.Scanning rate"=w266:dbl, "DAQParams.Average"=w265:dbl, "DAQParams.Sampling rate"=w264:dbl)
        n66 = Unbundle By Name(w235) -> ("SP->power Matrix"=w246:T7)
        n67 = Build Array(w267, w266, w265, w264) -> (w263:dbl[])
        n68 = To Long Integer(number=w263) -> (32bit integer=w262:i32[])
        n69 = for {
          tunnel: w262 -> [w344] mode=indexing
          tunnel: w303 -> [w345]
          tunnel: w302 -> [w343] mode=indexing
          shift-right: [w341] -> w301
          shift-left: w304 -> [w342]
          shift-right: [w339] -> w300
          shift-left: w305 -> [w340]
          n70 = call <vilib>:"Write Key (I32).vi"("section"=w345, "error in (no error)"=w340, "value"=w344, "key"=w343, "refnum"=w342) -> ("error out"=w339:errorcluster, "refnum out"=w341:T8)  [unwired: 4 in, 1 out]
        }
        n71 = Unbundle By Name(w235) -> ("z bead lookup table.z signal"=w252:dbl[], "z bead lookup table.z bead"=w251:dbl[])
        n72 = Index Array(array=w246, index (row) #1=0 ("index (row)"), index (row) #2=1 ("index (row)")) -> (element #1=w243:dbl[], element #2=w242:dbl[])  [unwired: 2 in]
        n73 = Unbundle By Name(w235) -> ("Z bead polynomial coeffs"=w261:dbl[])
        n74 = Build Array (concatenate)(w243, w242) -> (w241:dbl[])
        n75 = for {
          tunnel: w241 -> [w338] mode=indexing
          tunnel: w298 -> [w333]
          tunnel: w299 -> [w332] mode=indexing
          shift-right: [w334] -> w297
          shift-left: w301 -> [w336]
          shift-right: [w335] -> w296
          shift-left: w300 -> [w337]
          n76 = call-poly <vilib>:"Write Key.vi"("section"=w333, "error in (no error)"=w337, "value"=w338, "key"=w332, "refnum"=w336) -> ("error out"=w335:errorcluster, "refnum out"=w334:T8)  [unwired: 4 in, 1 out]
        }
        n77 = for {
          tunnel: w261 -> [w331] mode=indexing
          tunnel: w295 -> [w326]
          tunnel: w294 -> [w325] mode=indexing
          shift-right: [w327] -> w257
          shift-left: w297 -> [w329]
          shift-right: [w328] -> w260
          shift-left: w296 -> [w330]
          n78 = call-poly <vilib>:"Write Key.vi"("section"=w326, "error in (no error)"=w330, "value"=w331, "key"=w325, "refnum"=w329) -> ("error out"=w328:errorcluster, "refnum out"=w327:T8)  [unwired: 4 in, 1 out]
        }
        n79 = Build Array(w252, w251) -> (w250:dbl[][])
        n80 = Transpose 2D Array(2D array=w250) -> (transposed array=w249:dbl[][])
        n81 = Array To Spreadsheet String(delimiter (Tab)="\t" ("delimiter (\\t)"), array=w249, 3:"%.6e" ("format (%.3f)")) -> (spreadsheet string=w248:string)
        n82 = for {
          N: 1 -> [_]
          tunnel: w248 -> [w318]
          tunnel: w256 -> [w320]
          tunnel: w255 -> [w319] mode=indexing
          shift-right: [w321] -> w258
          shift-left: w257 -> [w323]
          shift-right: [w322] -> w259
          shift-left: w260 -> [w324]
          n83 = call-poly <vilib>:"Write Key.vi"("write raw string? (F)"=FALSE, "section"=w320, "error in (no error)"=w324, "value"=w318, "key"=w319, "refnum"=w323) -> ("error out"=w322:errorcluster, "refnum out"=w321:T8)  [unwired: 3 in, 1 out]
        }
        n84 = call <vilib>:"Close Config Data.vi"("error in (no error)"=w259, "refnum"=w258) -> ("error out"=w312:errorcluster, "file path"=w293:path)  [unwired: 8 in]
      }
      frame 3 {
        # "Unfinished yet"
        n85 = call <vilib>:"Open Config Data (compatibility).vi"("error in (no error)"=w410, "configuration file path"=w411) -> ("error out"=w409:errorcluster, "refnum"=w408:T8)  [unwired: 7 in, 1 out]
        n86 = for {
          tunnel: w383 -> [w461] mode=indexing
          tunnel: w406 -> [w456]
          tunnel: w405 -> [w455] mode=indexing
          shift-right: [w457] -> w404
          shift-left: w408 -> [w459]
          shift-right: [w458] -> w403
          shift-left: w409 -> [w460]
          n87 = call-poly <vilib>:"Write Key.vi"("section"=w456, "error in (no error)"=w460, "value"=w461, "key"=w455, "refnum"=w459) -> ("error out"=w458:errorcluster, "refnum out"=w457:T8)  [unwired: 4 in, 1 out]
        }
        n88 = for {
          tunnel: w382 -> [w454] mode=indexing
          tunnel: w401 -> [w449]
          tunnel: w402 -> [w448] mode=indexing
          shift-right: [w450] -> w399
          shift-left: w404 -> [w452]
          shift-right: [w451] -> w400
          shift-left: w403 -> [w453]
          n89 = call-poly <vilib>:"Write Key.vi"("section"=w449, "error in (no error)"=w453, "value"=w454, "key"=w448, "refnum"=w452) -> ("error out"=w451:errorcluster, "refnum out"=w450:T8)  [unwired: 4 in, 1 out]
        }
        n90 = for {
          tunnel: w381 -> [w447] mode=indexing
          tunnel: w397 -> [w442]
          tunnel: w398 -> [w441] mode=indexing
          shift-right: [w443] -> w395
          shift-left: w399 -> [w445]
          shift-right: [w444] -> w396
          shift-left: w400 -> [w446]
          n91 = call-poly <vilib>:"Write Key.vi"("section"=w442, "error in (no error)"=w446, "value"=w447, "key"=w441, "refnum"=w445) -> ("error out"=w444:errorcluster, "refnum out"=w443:T8)  [unwired: 4 in, 1 out]
        }
        n92 = for {
          tunnel: w380 -> [w439] mode=indexing
          tunnel: w394 -> [w440]
          tunnel: w393 -> [w438] mode=indexing
          shift-right: [w436] -> w392
          shift-left: w395 -> [w437]
          shift-right: [w434] -> w391
          shift-left: w396 -> [w435]
          n93 = call <vilib>:"Write Key (I32).vi"("section"=w440, "error in (no error)"=w435, "value"=w439, "key"=w438, "refnum"=w437) -> ("error out"=w434:errorcluster, "refnum out"=w436:T8)  [unwired: 4 in, 1 out]
        }
        n94 = for {
          tunnel: w379 -> [w433] mode=indexing
          tunnel: w389 -> [w428]
          tunnel: w390 -> [w427] mode=indexing
          shift-right: [w429] -> w388
          shift-left: w392 -> [w431]
          shift-right: [w430] -> w387
          shift-left: w391 -> [w432]
          n95 = call-poly <vilib>:"Write Key.vi"("section"=w428, "error in (no error)"=w432, "value"=w433, "key"=w427, "refnum"=w431) -> ("error out"=w430:errorcluster, "refnum out"=w429:T8)  [unwired: 4 in, 1 out]
        }
        n96 = for {
          tunnel: w378 -> [w426] mode=indexing
          tunnel: w386 -> [w421]
          tunnel: w385 -> [w420] mode=indexing
          shift-right: [w422] -> w377
          shift-left: w388 -> [w424]
          shift-right: [w423] -> w376
          shift-left: w387 -> [w425]
          n97 = call-poly <vilib>:"Write Key.vi"("section"=w421, "error in (no error)"=w425, "value"=w426, "key"=w420, "refnum"=w424) -> ("error out"=w423:errorcluster, "refnum out"=w422:T8)  [unwired: 4 in, 1 out]
        }
        n98 = Array To Spreadsheet String(delimiter (Tab)="\t" ("delimiter (\\t)"), array=w369, 3:"%.6e" ("format (%.3f)")) -> (spreadsheet string=w368:string)
        n99 = for {
          N: 1 -> [_]
          tunnel: w368 -> [w413]
          tunnel: w373 -> [w415]
          tunnel: w372 -> [w414] mode=indexing
          shift-right: [w416] -> w374
          shift-left: w377 -> [w418]
          shift-right: [w417] -> w375
          shift-left: w376 -> [w419]
          n100 = call-poly <vilib>:"Write Key.vi"("write raw string? (F)"=FALSE, "section"=w415, "error in (no error)"=w419, "value"=w413, "key"=w414, "refnum"=w418) -> ("error out"=w417:errorcluster, "refnum out"=w416:T8)  [unwired: 3 in, 1 out]
        }
        n101 = call <vilib>:"Close Config Data.vi"("error in (no error)"=w375, "refnum"=w374) -> ("error out"=w407:errorcluster, "file path"=w384:path)  [unwired: 8 in]
      }
      frame 2 {
        n102 = call <vilib>:"Check if File or Folder Exists.vi"("path"=w463) -> ("file or folder exists?"=w462:bool)  [unwired: 8 in, 2 out]
        n103 = case shown="False" w462 {
          tunnel: w468 -> [w474 _]
          tunnel: [w473 w476] -> w467
          tunnel: w466 -> [w472 w475]
          tunnel: [w471 w475] -> w465
          tunnel: w463 -> [w469 w476]
          frame False {
            n104 = Copy(8:w472, 9:TRUE ("overwrite (F)"), 10:w469, 11:w474) -> (0:w471:errorcluster, 3:w473:path)  [unwired: 1 in, 1 out]
          }
          frame True {
          }
        }
        n105 = call <vilib>:"Clear Errors.vi"("error in (no error)"=w465) -> ("error out"=w464:errorcluster)  [unwired: 5 in, 1 out]
      }
    }
  }
  "error out" <- w33
  "file path out" <- w32
  "Params out" <- w1
  n106 = To Variant(anything="Params in") -> (Variant=w29:variant)
  n107 = To Variant(anything=w1) -> (Variant=w28:variant)
  n108 = Equal?(x=w29, y=w28) -> (x = y?=→"succeeded in writing to ini file ?":bool)
  n109 = local write "Params in"(w1) -> ()
